vi "Read TestInfo.vi"(8 "error in (no error)":errorcluster, 11 "TestMeasureStep in":refnum<class "TestMeasureStep.lvclass">) -> (0 "error out":errorcluster, 2 "TestInfo 2":T1, 3 "TestMeasureStep out":refnum<class "TestMeasureStep.lvclass">)   [LabVIEW 2017, in "TestMeasureStep.lvclass"]
uses:
  TestMeasureStep.lvclass
  TypeDef/TesstepType.ctl
  testSeq/Typedef/TestStatus.ctl
  TestMeasureStep.lvclass/TestMeasureStep.ctl
  testSeq/TestSeqClass.lvclass
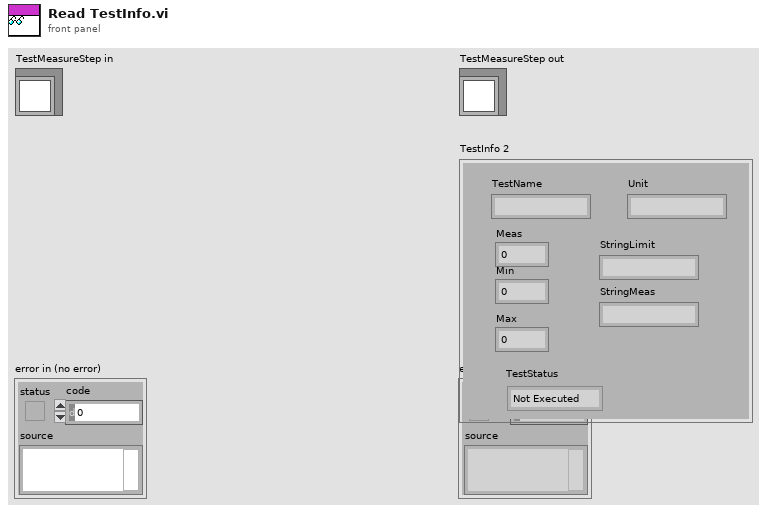
[diagram p1: front panel]
types:
  T1 = typedef "TestSeqClass.lvclass/TesstepType.ctl" = cluster{"TestName":string, "Meas":dbl, "Min ":dbl, "Max":dbl, "TestStatus":T2, "StringLimit":string, "StringMeas":string, "Unit":string}
  T2 = typedef "TestStatus.ctl" = enum16{"Not Executed", "Passed", "Failed", "Inconclusive", "Processing"}
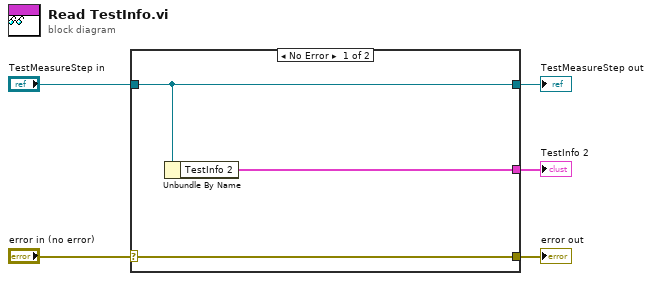
[diagram p0: block diagram]
diagram:
  n1 = case shown="No Error" "error in (no error)" {
    selector: "error in (no error)" -> [w8 w9]
    tunnel: [w8 w9] -> w4
    tunnel: [w7 w10] -> w2
    tunnel: "TestMeasureStep in" -> [w7 w10]
    tunnel: [w6 _] -> w1
    frame No Error {
      n2 = Unbundle By Name(w7) -> ("TestInfo 2"=w6:T1)
    }
    frame Error {
    }
  }
  "error out" <- w4
  "TestMeasureStep out" <- w2
  "TestInfo 2" <- w1
